vi "ms_to_Time.vi"(11 "TimeOut[ms]":i32) -> (3 "Time[String]":string)   [LabVIEW 2021, in "Time.lvlib"]
uses:
  Time.lvlib
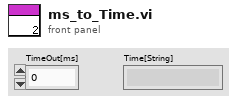
[diagram p1: front panel]
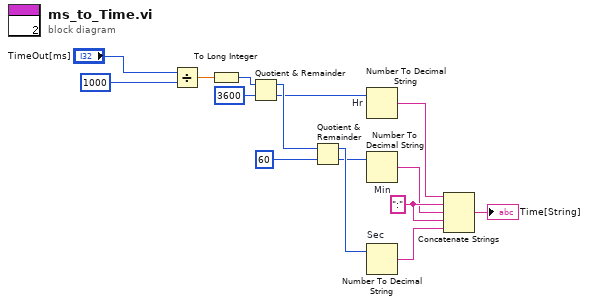
[diagram p0: block diagram]
diagram:
  w9 = ":" ("string")
  n1 = Divide(x="TimeOut[ms]", y=1000) -> (x/y=w14:dbl)
  n2 = To Long Integer(number=w14) -> (32bit integer=w15:i32)
  n3 = Quotient & Remainder(x=w15, y=3600) -> (x-y*floor(x/y)=w3:i32, floor(x/y)=w2:i32)
  n4 = Quotient & Remainder(x=w3, y=60) -> (x-y*floor(x/y)=w6:i32, floor(x/y)=w5:i32)
  n5 = Number To Decimal String "Hr"(number=w2) -> (decimal integer string=w7:string)  [unwired: 1 in]
  n6 = Number To Decimal String "Min"(number=w5) -> (decimal integer string=w8:string)  [unwired: 1 in]
  n7 = Number To Decimal String "Sec"(number=w6) -> (decimal integer string=w10:string)  [unwired: 1 in]
  n8 = Concatenate Strings(w7, w9, w8, w9, w10) -> (→"Time[String]":string)
